vi "restartBuffer.vi"(8 "error in (no error)":errorcluster, 11 "ElectrometerController in":refnum<class "ElectrometerController.lvclass">) -> (0 "error out":errorcluster, 3 "ElectrometerController out":refnum<class "ElectrometerController.lvclass">)   [LabVIEW 2016, in "ElectrometerController.lvclass"]
uses:
  ElectrometerController.lvclass
  Electrometer/Electrometer.lvclass
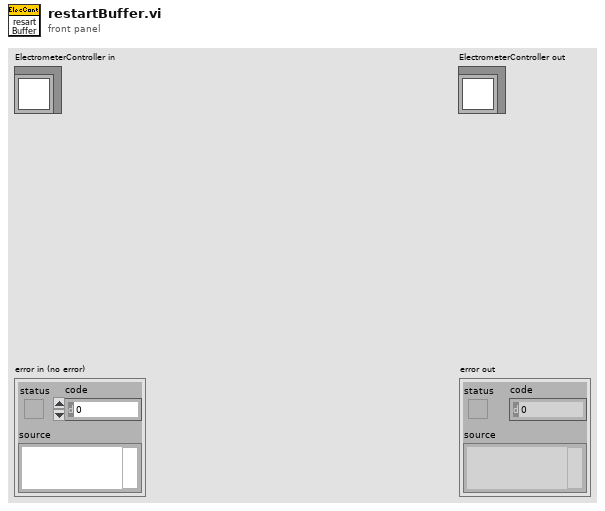
[diagram p1: front panel]
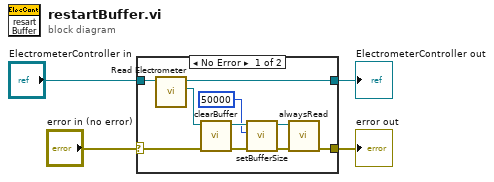
[diagram p0: block diagram]
diagram:
  n1 = case shown="No Error" "error in (no error)" {
    selector: "error in (no error)" -> [w11 w16]
    tunnel: [w10 w16] -> w3
    tunnel: [w13 w15] -> w1
    tunnel: "ElectrometerController in" -> [w14 w15]
    frame No Error {
      n2 = call-dynamic "Read Electrometer.vi"("ElectrometerController in"=w14) -> ("Electrometer.lvclass"=w12:refnum<class "Electrometer.lvclass">, "ElectrometerController out"=w13:refnum<class "ElectrometerController.lvclass">)  [unwired: 8 in, 1 out]
      n3 = call "clearBuffer.vi"("error in (no error)"=w11, "Electrometer in"=w12) -> ("error out"=w9:errorcluster, "Electrometer out"=w8:refnum<class "Electrometer.lvclass">)  [unwired: 8 in]
      n4 = call "setBufferSize.vi"("error in (no error)"=w9, "bufferSize"=u32 50000, "Electrometer in"=w8) -> ("error out"=w5:errorcluster, "Electrometer out"=w6:refnum<class "Electrometer.lvclass">)  [unwired: 7 in]
      n5 = call "alwaysRead.vi"("error in (no error)"=w5, "Electrometer in"=w6) -> ("error out"=w10:errorcluster)  [unwired: 8 in, 1 out]
    }
    frame Error {
    }
  }
  "error out" <- w3
  "ElectrometerController out" <- w1
